vi "write.vi"(0 "object in":refnum<class "MBinteractive.lvclass">, 1 "starting address":u16 caption="起始地址", 2 "holding register values":u16[](array[numeric]) caption="写入保持寄存器的值", 5 "error in (no error)":errorcluster) -> (14 "object out":refnum<class "MBinteractive.lvclass">, 19 "error out":errorcluster)   [LabVIEW 2016, in "MBinteractive.lvclass"]
uses:
  MBinteractive.lvclass
  MBinteractive.lvclass/MBinteractive.ctl
  <vilib>/NI/Modbus Library/API/Modbus API.lvclass
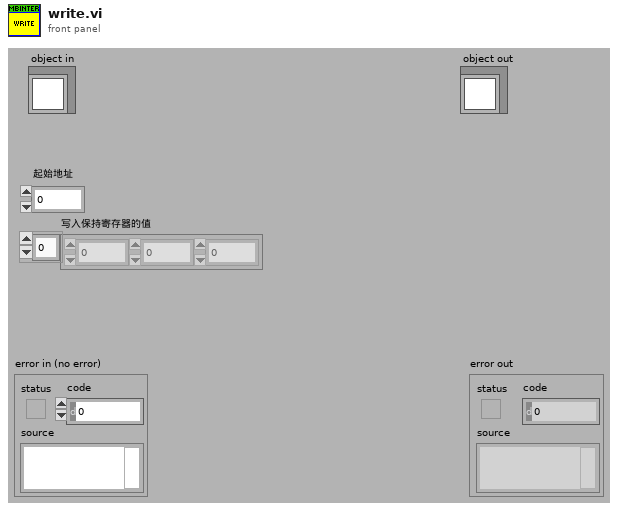
[diagram p1: front panel]
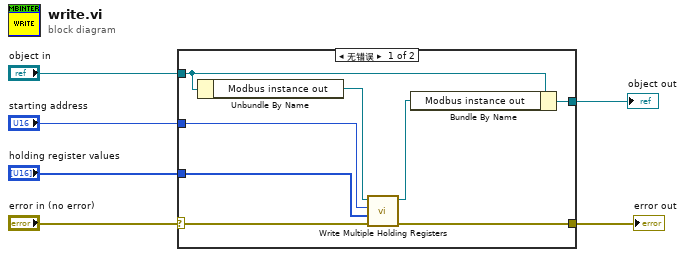
[diagram p0: block diagram]
diagram:
  n1 = case shown="无错误" "error in (no error)" {
    selector: "error in (no error)" -> [w9 w16]
    tunnel: [w8 w16] -> w5
    tunnel: [w13 w15] -> w3
    tunnel: "object in" -> [w14 w15]
    tunnel: "starting address" -> [w11 _]
    tunnel: "holding register values" -> [w10 _]
    frame No Error {
      n2 = Unbundle By Name(w14) -> ("Modbus instance out"=w12:refnum<class "Modbus API.lvclass">)
      n3 = call-dynamic "Write Multiple Holding Registers.vi"("error in"=w9, "registers to write"=w10, "starting address"=w11, "Modbus instance in"=w12) -> ("error out"=w8:errorcluster, "Modbus instance out"=w7:refnum<class "Modbus API.lvclass">)  [unwired: 6 in]
      n4 = Bundle By Name(cluster=w14, "Modbus instance out"=w7) -> (w13:refnum<class "MBinteractive.lvclass">)
    }
    frame Error {
    }
  }
  "error out" <- w5
  "object out" <- w3
